vi "Clone Subtree.vi"(8 "error in (no error)":errorcluster, 9 "Array Index (None)":i32=-1, 10 "Hierarchy":string[](array[string]), 11 "Value Tree in":refnum<class "Value Tree.lvclass">) -> (0 "error out":errorcluster, 2 "Subtree":refnum<class "Value Tree.lvclass">, 3 "Value Tree out":refnum<class "Value Tree.lvclass">)   [LabVIEW 2020, in "HTTP Server.lvlib" / "Value Tree.lvclass"]
uses:
  Value Tree.lvclass
  Value Tree.lvclass/Value Tree.ctl
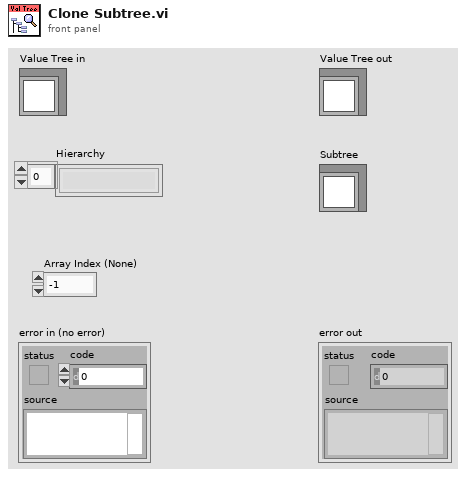
[diagram p1: front panel]
types:
  T1 = typedef "HTTP Server.lvlib/Value Tree.lvclass/Local Info.ctl" = cluster{"Type":T2, "Value":string, "Children":string[], "Size":i32}
  T2 = typedef "HTTP Server.lvlib/Value Tree.lvclass/Local Type.ctl" = enum16{"Scalar", "Object", "Array"}
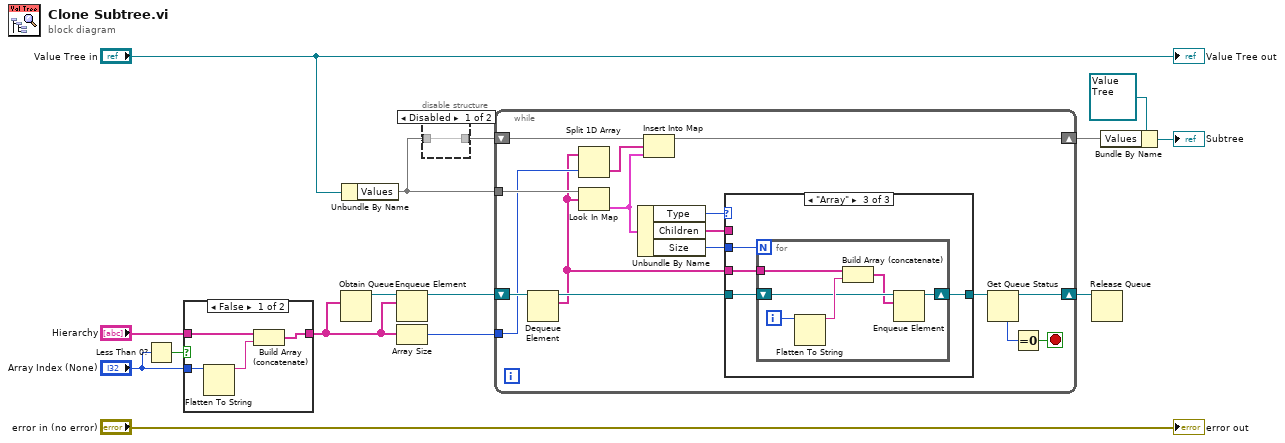
[diagram p0: block diagram]
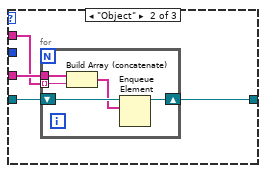
[diagram p5: hidden frame]
diagram:
  n1 = Less Than 0?(x="Array Index (None)") -> (x < 0?=w4:bool)
  n2 = case shown="False" w4 {
    tunnel: [w16 w20] -> w3
    tunnel: "Hierarchy" -> [w18 w20]
    tunnel: "Array Index (None)" -> [w19 _]
    frame False {
      n3 = Flatten To String(anything=w19) -> (data string=w17:string)  [unwired: 3 in, 2 out]
      n4 = Build Array (concatenate)(w18, w17) -> (w16:string[])
    }
    frame True {
    }
  }
  n5 = Obtain Queue(element data type=w3) -> (queue out=w13:refnum<queue>)  [unwired: 4 in, 2 out]
  n6 = Unbundle By Name("Value Tree in") -> ("Values"=w9:map{string[], T1})
  n7 = Enqueue Element(queue=w13, element=w3) -> (queue out=w12:refnum<queue>)  [unwired: 2 in, 2 out]
  n8 = Array Size(array=w3) -> (size(s)=w11:i32)
  n9 = disable-structure shown="Disabled" {
    disable-tunnel: [w21 _] -> w10
    disable-tunnel: w9 -> [w21 _]
    frame Disabled {
    }
    frame Enabled {
    }
  }
  n10 = while {
    shift-right: [w35] -> w8
    shift-left: w12 -> [w37]
    tunnel: w9 -> [w36]
    tunnel: w11 -> [w32]
    shift-right: [w23] -> w5
    shift-left: w10 -> [w31]
    stop <- w33 stop-if-true
    n11 = Dequeue Element(queue=w37) -> (queue out=w27:refnum<queue>, element=w25:string[])  [unwired: 2 in, 2 out]
    n12 = Split 1D Array(array=w25, index=w32) -> (second subarray=w30:string[])  [unwired: 1 out]
    n13 = Look In Map(map=w36, key=w25) -> (value=w29:T1)  [unwired: 1 in, 1 out]
    n14 = Unbundle By Name(w29) -> ("Type"=w28:T2, "Children"=w26:string[], "Size"=w24:i32)
    n15 = Insert Into Map(map in=w31, key=w30, value=w29) -> (map out=w23:map{string[], T1})  [unwired: 2 out]
    n16 = case shown="\"Array\"" w28 {
      tunnel: w27 -> [w38 w40 w49]
      tunnel: w26 -> [_ w41 _]
      tunnel: w25 -> [_ w42 w50]
      tunnel: w24 -> [_ _ w51]
      tunnel: [w38 w39 w48] -> w22
      frame "Scalar" {
      }
      frame "Object" {
        n17 = for {
          tunnel: w42 -> [w47]
          tunnel: w41 -> [w46] mode=indexing
          shift-right: [w43] -> w39
          shift-left: w40 -> [w45]
          n18 = Build Array (concatenate)(w47, w46) -> (w44:string[])
          n19 = Enqueue Element(queue=w45, element=w44) -> (queue out=w43:refnum<queue>)  [unwired: 2 in, 2 out]
        }
      }
      frame "Array" {
        n20 = for {
          N: w51 -> [_]
          tunnel: w50 -> [w56]
          shift-right: [w52] -> w48
          shift-left: w49 -> [w54]
          i -> [w57]
          n21 = Flatten To String(anything=w57) -> (data string=w55:string)  [unwired: 3 in, 2 out]
          n22 = Build Array (concatenate)(w56, w55) -> (w53:string[])
          n23 = Enqueue Element(queue=w54, element=w53) -> (queue out=w52:refnum<queue>)  [unwired: 2 in, 2 out]
        }
      }
    }
    n24 = Get Queue Status(queue=w22) -> (queue out=w35:refnum<queue>, # elements in queue=w34:i32)  [unwired: 2 in, 6 out]
    n25 = Equal To 0?(x=w34) -> (x = 0?=w33:bool)
  }
  n26 = Release Queue(queue=w8) -> ()  [unwired: 2 in, 3 out]
  n27 = Bundle By Name(cluster=refnum<class "Value Tree.lvclass"> refnum ("Subtree"), "Values"=w5) -> (→"Subtree":refnum<class "Value Tree.lvclass">)
  "error out" <- "error in (no error)"
  "Value Tree out" <- "Value Tree in"
